vi "Detect Text (ARGB).vi"(8 "error in (no error)":errorcluster, 10 "ARGB Image in":T4, 11 "Text Detector in":refnum<class "Text Detector.lvclass">) -> (0 "error out":errorcluster, 2 "Detections":T1[](array[typedef]), 3 "Text Detector":refnum<class "Text Detector.lvclass">)   [LabVIEW 2020, in "feature_detection.lvlib" / "Text Detector.lvclass"]
uses:
  Text Detector.lvclass
  Text Detector.lvclass/Text Detector.ctl
  eed31af3-93fd-418d-8fe9-3dec6e1d7c5b.vi
  image/ARGB Image.ctl
  image/image.lvlib
  common/Image Point (Float).ctl
  common/common.lvlib
  common/Quad Corners.ctl
  Detection.ctl
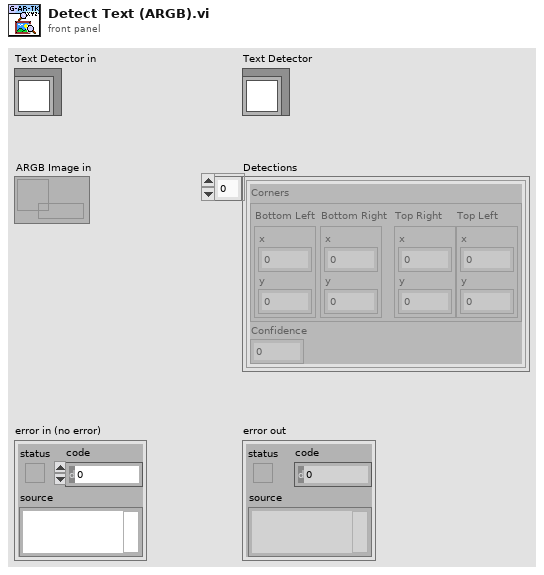
[diagram p1: front panel]
types:
  T1 = typedef "feature_detection.lvlib/Text Detector.lvclass/Detection.ctl" = cluster{"Corners":T2, "Confidence":sgl}
  T2 = typedef "common.lvlib/Quad Corners.ctl" = cluster{"Bottom Left":T3, "Bottom Right":T3, "Top Right":T3, "Top Left":T3}
  T3 = typedef "common.lvlib/Image Point (Float).ctl" = cluster{"x":dbl, "y":dbl}
  T4 = typedef "image.lvlib/ARGB Image.ctl" = refnum<data-value>
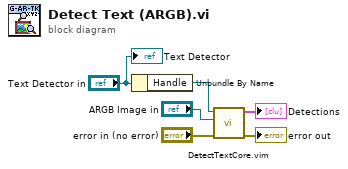
[diagram p0: block diagram]
diagram:
  n1 = Unbundle By Name("Text Detector in") -> ("Handle"=w5:refnum<data-value>)
  n2 = call "DetectTextCore.vim"("error in (no error)"="error in (no error)", "Greyscale Image in"="ARGB Image in", "Detector in"=w5) -> ("error out"=→"error out":errorcluster, "Detections"=→"Detections":T1[])  [unwired: 7 in]
  "Text Detector" <- "Text Detector in"
